vi "Channel group helper.vi"(8 "Pos/Vel":enum16{"Position", "Velocity"}(ring)=enum."Velocity", 9 "Eye component":enum16{"x", "y", "z"}(ring)=enum."z", 10 "Eye":enum16{"Right", "Left"}(ring)=enum."Left", 11 "Channel Groups":i32[][][](array[numeric])) -> (3 "Channel":i32)   [LabVIEW 2013]
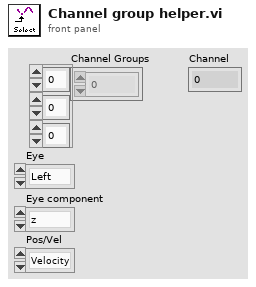
[diagram p1: front panel]
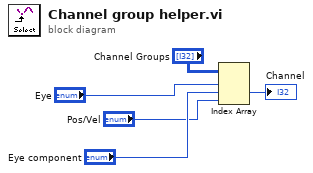
[diagram p0: block diagram]
diagram:
  n1 = Index Array(array="Channel Groups", index (dim 0)="Eye", index (dim 1)="Eye component", index (dim 2)="Pos/Vel") -> (element=→"Channel":i32)
